vi "1 - DAQmx Bus Digital Input.vi"() -> ()   [LabVIEW 2021]
uses:
  <vilib>/TSA/Omni-Bus/Omni-Bus/Omni_Bus.lvclass
  <vilib>/TSA/Omni-Bus/Omni-Bus/Support/Broad Types.ctl
  <vilib>/TSA/Abstract Data Classes/Abs_Types/Type/Abs_Type.lvclass/Abs_Type.ctl
  <vilib>/TSA/Omni-Bus/Omni-Bus/Omni_Bus.lvclass/Omni_Bus.ctl
  <vilib>/TSA/Omni-Bus/Omni-Bus/Support/Read/Read Boolean.vi
  <vilib>/TSA/Omni-Bus/Omni-Bus/Support/FindVar.vi
  <vilib>/Utility/error.llb/Clear Errors.vi
  <vilib>/TSA/Omni-Bus/Omni-Bus/Properties/Read Var Map.vi
  <vilib>/TSA/Abstract Data Classes/Abs_Types/Type/Properties/Read Tag.vi
  DAQmx-Bus.lvclass
  C:/Program Files (x86)/National Instruments/LabVIEW 2021/vi.lib/TSA/Omni-Bus/Omni-Bus/Bus Access/Bus_Access.lvclass
  <vilib>/TSA/Abstract Data Classes/Abs_Types/Boolean/Abs_Boolean.lvclass
  C:/Program Files (x86)/National Instruments/LabVIEW 2021/vi.lib/TSA/Abstract Data Classes/Abs_Types/Type/Abs_Type.lvclass
  <vilib>/TSA/Abstract Data Classes/Abs_Types/Value/Abs_Value.lvclass
  <vilib>/TSA/Omni-Bus/Omni-Bus/Support/Check For Read Only Error.vi
  <vilib>/TSA/Omni-Bus/Omni-Bus/Support/Incorrect Tag String Error.vi
  <vilib>/TSA/Abstract Data Classes/Abs_Types/Type/Abs_Type.lvclass
panel:
  in  "DAQmx Digital Input Task":refnum<k21>="Digital Input"
  out "Boolean":bool
  in  "stop":bool
  in  "Digital Input Tag":string(combo)
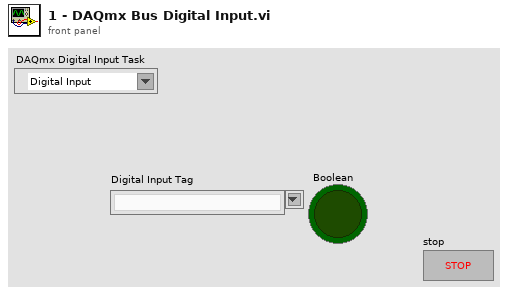
[diagram p1: front panel]
types:
  T1 = typedef "Omni_Bus.lvclass/Broad Types.ctl" = enum16{"All Tags", "NI Specific Type", "Boolean", "String", "Numeric", "Float", "Integer", "Collection", "All Value Types", "Non Value Types"}
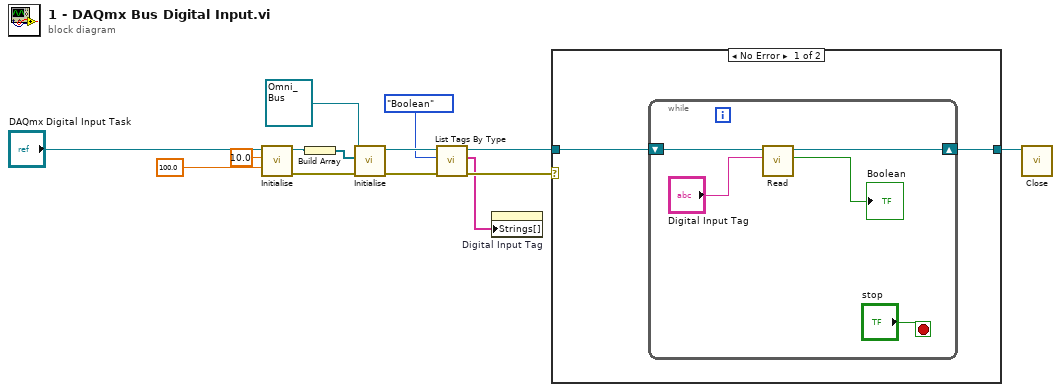
[diagram p0: block diagram]
diagram:
  n1 = call "Initialise.vi"("Update Rate (Hz) - Non HW Timed"=100.0, "timeout (s)"=10.0 ("timeout"), "DAQmx Task"="DAQmx Digital Input Task") -> ("error out"=w10:errorcluster, "DAQmx-Bus out"=w2:refnum<class "DAQmx-Bus.lvclass">)  [unwired: 7 in]
  n2 = Build Array(w2) -> (w12:refnum<class "DAQmx-Bus.lvclass">[])
  n3 = call-dynamic "Initialise.vi"("error in (no error)"=w10, "Bus Access"=w12, "Var Bus in"=refnum<class "Omni_Bus.lvclass"> refnum) -> ("error out"=w7:errorcluster, "Var Bus out"=w8:refnum<class "Omni_Bus.lvclass">)  [unwired: 7 in]
  n4 = call <vilib>:"List Tags By Type.vi"("error in (no error)"=w7, "Broad Types"=Broad_Types."Boolean", "Var Bus in"=w8) -> ("error out"=w5:errorcluster, "Tags"=w4:string[], "Var Bus out"=w6:refnum<class "Omni_Bus.lvclass">)  [unwired: 5 in, 1 out]
  n5 = property on="Digital Input Tag" class="CmbBox"("Strings[]"=w4) -> ()  [unwired: 2 in, 2 out]
  n6 = case shown="No Error" w5 {
    tunnel: [w16 w22] -> w9
    tunnel: w6 -> [w15 w22]
    frame No Error {
      n7 = while {
        shift-right: [w21] -> w16
        shift-left: w15 -> [w20]
        stop <- "stop" stop-if-true
        n8 = call-poly <vilib>:"Read.vi"("Tag"="Digital Input Tag", "Var Bus in"=w20) -> ("Boolean"=→"Boolean":bool, "Var Bus out"=w21:refnum<class "Omni_Bus.lvclass">)  [unwired: 7 in, 1 out]
      }
    }
    frame Error {
    }
  }
  n9 = call-dynamic "Close.vi"("Data in"=w9) -> ()  [unwired: 9 in, 2 out]
